vi "UsrProfiles-Update user profiles list.vi"(8 "error in":errorcluster) -> (0 "error out":errorcluster)   [LabVIEW 2013]
uses:
  Typedefs/Save-Load enum.ctl
  Globals/gl_UsrProfiles globals.vi
  Global Variables/General Globals.vi
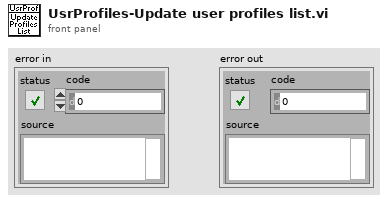
[diagram p1: front panel]
types:
  T1 = typedef "User login window refs.ctl" = cluster{"User profiles window ref":refnum<k9>, "Users listbox":refnum<vi>, "Profiles listbox":refnum<vi>, "Last used":refnum<vi>}
  T2 = typedef "Save-Load enum.ctl" = enum16{"Save to file", "Load from file", "Compare from file"}
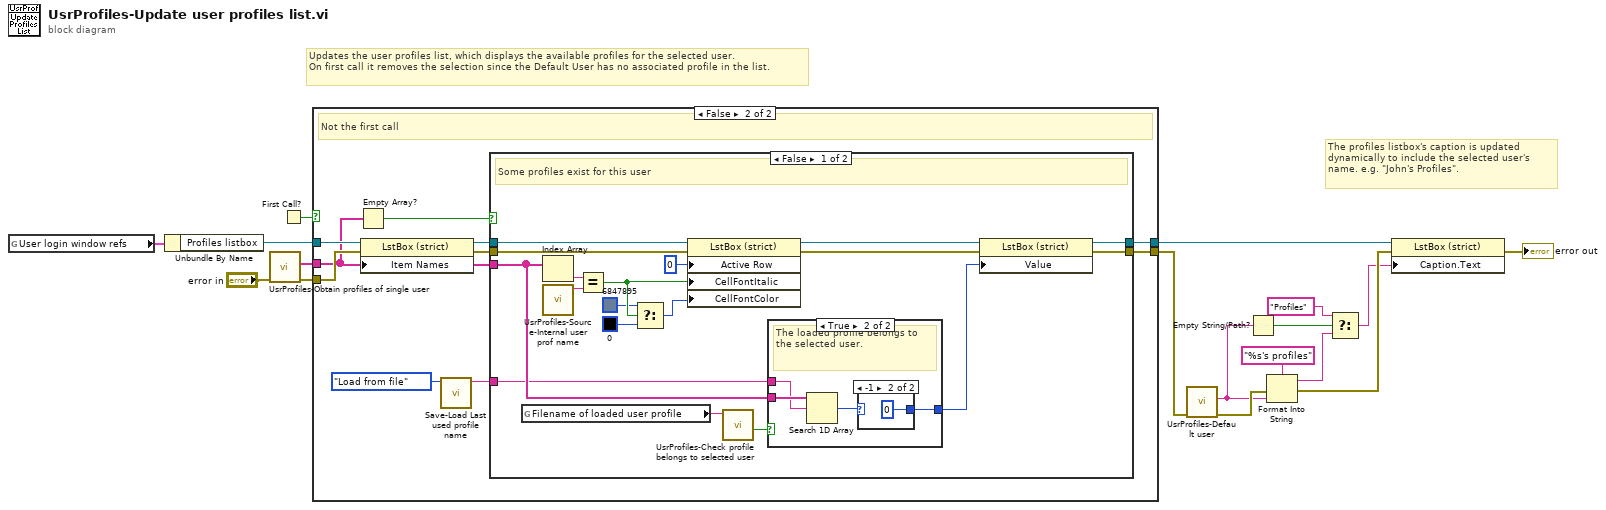
[diagram p0: block diagram]
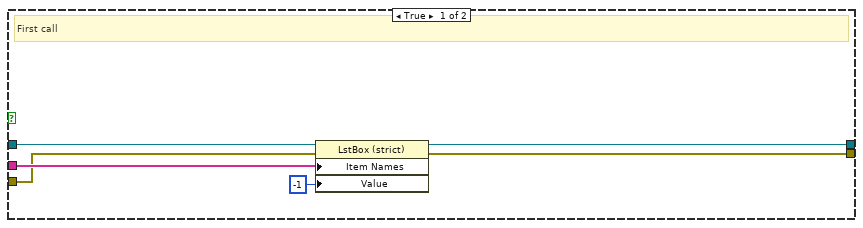
[diagram p2: hidden frame]
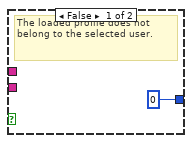
[diagram p3: hidden frame]
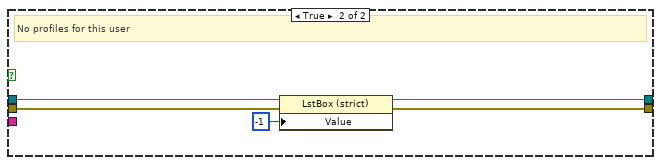
[diagram p5: hidden frame]
diagram:
  # "The profiles listbox's caption is updated dynamically to include the selected user's name. e.g. \"John's Profiles\"."
  # "Updates the user profiles list, which displays the available profiles for the selected user.\nOn first call it removes the selection since the Default User has no associated profile in the list."
  n1 = global read "gl_UsrProfiles globals.vi" "User login window refs"() -> (w14:T1)
  n2 = Unbundle By Name(w14) -> ("Profiles listbox"=w16:refnum<vi>)
  n3 = call "UsrProfiles-Obtain profiles of single user.vi"("error in"="error in") -> ("error out"=w13:errorcluster, "User profile names"=w15:string[])  [unwired: 9 in]
  n4 = First Call?() -> (First Call?: T/F=w17:bool)
  n5 = case shown="False" w17 {
    tunnel: w15 -> [w23 w27]
    tunnel: w16 -> [w22 w33]
    tunnel: [w21 w30] -> w1
    tunnel: w13 -> [w20 w32]
    tunnel: [w18 w25] -> w4
    frame True {
      # "First call"
      n6 = property on="Property Node" class="LstBox (strict)"(reference=w22, error in=w20, "Item Names"=w23, "Value"=-1) -> (reference out=w18:refnum<vi>, error out=w21:errorcluster)
    }
    frame False {
      # "Not the first call"
      n7 = Empty Array?(array=w27) -> (empty?=w28:bool)
      n8 = property on="Property Node" class="LstBox (strict)"(reference=w33, error in=w32, "Item Names"=w27) -> (reference out=w29:refnum<vi>, error out=w31:errorcluster)
      n9 = call "Save-Load Last used profile name.vi"("Function"=Save-Load_enum."Load from file") -> ("Last used profile for selected user"=w26:string)  [unwired: 8 in, 2 out]
      n10 = case shown="False" w28 {
        tunnel: w31 -> [w49 w63]
        tunnel: [w50 w62] -> w30
        tunnel: w29 -> [w51 w61]
        tunnel: w27 -> [w48 _]
        tunnel: w26 -> [w47 _]
        tunnel: [w46 w59] -> w25
        frame False {
          # "Some profiles exist for this user"
          n11 = global read "General Globals.vi" "Filename of loaded user profile"() -> (w36:string)
          n12 = Index Array(array=w48) -> (element=w44:string)  [unwired: 1 in]
          n13 = call "UsrProfiles-Source-Internal user prof name.vi"() -> ("Previous session profile name"=w43:string)  [unwired: 11 in]
          n14 = Equal?(x=w44, y=w43) -> (x = y?=w41:bool)
          n15 = Select(t=u32 6847895 ("Color Box"), s=w41, f=u32 0) -> (s? t:f=w39:u32)
          n16 = property on="Property Node" class="LstBox (strict)"(reference=w51, error in=w49, "Active Row"=0 ("index of element"), "CellFontItalic"=w41, "CellFontColor"=w39) -> (reference out=w38:refnum<vi>, error out=w37:errorcluster)
          n17 = call "UsrProfiles-Check profile belongs to selected user.vi"("Filename of loaded user profile"=w36) -> ("Belongs to selected user"=w35:bool)  [unwired: 10 in]
          n18 = case shown="True" w35 {
            tunnel: [0 w55] -> w34
            tunnel: w48 -> [_ w54]
            tunnel: w47 -> [_ w53]
            frame False {
              # "The loaded profile does not belong to the selected user."
            }
            frame True {
              # "The loaded profile belongs to the selected user."
              n19 = Search 1D Array(1D array=w54, element=w53) -> (index of element=w56:i32)  [unwired: 1 in]
              n20 = case shown="-1" w56 {
                selector: w56 -> [w57 _]
                tunnel: [w57 0] -> w55
                frame Default {
                }
                frame -1 {
                }
              }
            }
          }
          n21 = property on="Property Node" class="LstBox (strict)"(reference=w38, error in=w37, "Value"=w34) -> (reference out=w46:refnum<vi>, error out=w50:errorcluster)
        }
        frame True {
          # "No profiles for this user"
          n22 = property on="Property Node" class="LstBox (strict)"(reference=w61, error in=w63, "Value"=-1) -> (reference out=w59:refnum<vi>, error out=w62:errorcluster)
        }
      }
    }
  }
  n23 = call "UsrProfiles-Default user.vi"("error in (no error)"=w1) -> ("error out"=w3:errorcluster, "Selected user's name"=w2:string)  [unwired: 8 in, 1 out]
  n24 = Empty String/Path?(string/path=w2) -> (empty?=w9:bool)
  n25 = Format Into String(format string="%s's profiles", error in=w3, w2) -> (resulting string=w8:string, error out=w7:errorcluster)  [unwired: 1 in]
  n26 = Select(t="Profiles", s=w9, f=w8) -> (s? t:f=w6:string)
  n27 = property on="Property Node" class="LstBox (strict)"(reference=w4, error in=w7, "Caption.Text"=w6) -> (error out=→"error out":errorcluster)  [unwired: 1 out]
